vi "_SeqMgr.Code Test.vi"(11 "Module Config":T4={"Name"="SeqMgr_SW_Ver", "Parent Q"=refnum, "Is Child?"=FALSE, "Index"=0, "Dirs"={"Root"=path "", "Config"=path "C:/ATE/Config", "Logs"=path "C:/ATE/Logs", "Reports"=path "C:/ATE/Reports", "App Data"=path "C:/ProgramData/MAIN"}, "Simulate"=FALSE, "SimCtrl"=refnum}) -> ()   [LabVIEW 2024, in "EQMF.lvlib" / "SeqMgr.lvlib"]
uses:
  SeqMgr.lvlib
  SeqMgr.Result State Enum.ctl
  Module/Module Config.ctl
  Queues/Q.Element.ctl
  Module/Module.Working Dirs.ctl
  Module/Module.SW Version Info.ctl
  SeqMgr.Result Info.ctl
  Module/Window/Window.Task, Action.ctl
  Event Log/Log Action Class/Event Log.Log Params.ctl
  Event Log/Event Notification/Event Log.Log Level.ctl
  SeqMgr.lvclass
  SeqMgr.Progress Controls.ctl
  SeqMgr.Result Control Ref.ctl
  Config/Stored Controls/Class.SaveCtrls.lvclass
  Queues/Queue Utils.lvlib
  Module/Module Utils.lvlib
  Event Log/Event Log.lvlib
  Scheduler/Scheduler.lvlib
  Menu/Menu Utils.lvlib
  Config/Config Utils.lvlib
panel:
  in  "Main Tab":enum32{"Operate", "Maint"}(tab)
  in  "Default Delay ms":i32=100
  out "Simulate Indication":string="Simulating Instruments"
  out "Rev":string="v1.0.0"
  out "Test Ctrl Tab":enum32{"Idle", "Running", "Completed"}(tab)
  in  "Test Start":bool
  in  "SN":string
  out "UUT SN Status":string="Enter Operator and SN then click Start."
  out "Test Running":bool
  out "Progress":dbl(slide) scale=0.0..1.0
  in  "Test Abort":bool
  out "SN 2":string caption="SN"
  out "Failing Status":string="Failing"
  in  "Test Reset":bool
  out "SN 3":string caption="SN"
  out "Result":T2
  out "Start Time":timestamp
  out "Duration(s)":dbl format="%.2f"
  out "End Time":timestamp
  out "Current Step":string[](array[string])
  in  "Seq Steps":string[][](array[string])=[["Action1", "1000"], ["Action2", "100"], ["Action3", "500"], ["Action4", "500"]]
  out "Status":string
  in  "Stop on Fail":bool
  in  "Stop on Error":bool=TRUE
  out "Seq Name":string
  in  "Result Info":T3={"State"=enum."Passing", "Code"=0, "Description"=""}
  in  "Leave Maint":bool
  in  "SW Rev":T6={"AppName"="SeqMgr_SW_Ver", "Company"="KwestEng", "Version"="1.0", "Description"="", "PN"=""}
  # "Seq Test"
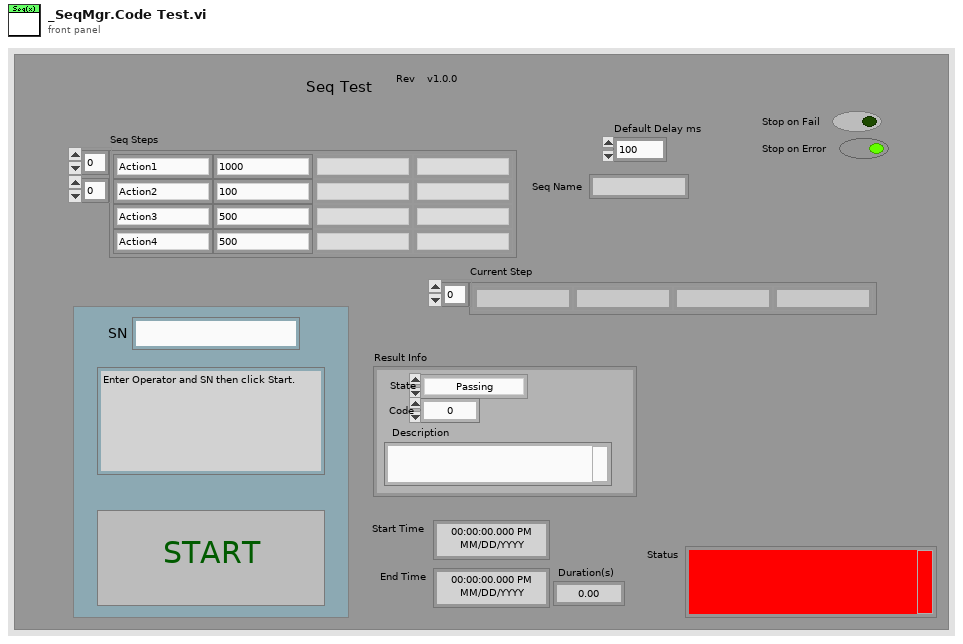
[diagram p1: front panel]
types:
  T1 = typedef "EQMF.lvlib/SeqMgr.lvlib/SeqMgr.Result State Enum.ctl" = enum16{"None", "Passing", "Failing", "PASS", "FAIL", "ABORT", "ERROR"}
  T2 = cluster{"State":T1, "Code":i32, "Description":string}
  T3 = typedef "EQMF.lvlib/SeqMgr.lvlib/SeqMgr.Result Info.ctl" = cluster{"State":T1, "Code":i32, "Description":string}
  T4 = typedef "EQMF.lvlib/Module Utils.lvlib/Module Config.ctl" = cluster{"Name":string, "Parent Q":refnum<queue>, "Is Child?":bool, "Index":i32, "Dirs":T5, "Simulate":bool, "SimCtrl":refnum<vi>}
  T5 = typedef "EQMF.lvlib/Module Utils.lvlib/Module.Working Dirs.ctl" = cluster{"Root":path, "Config":path, "Logs":path, "Reports":path, "App Data":path}
  T6 = typedef "EQMF.lvlib/Module Utils.lvlib/Module.SW Version Info.ctl" = cluster{"AppName":string, "Company":string, "Version":string, "Description":string, "PN":string}
  T7 = typedef "EQMF.lvlib/Module Utils.lvlib/Module Sys Info.ctl" = cluster{"Main Q":refnum<queue>, "Exe":bool, "SW Rev":T6, "Self Ref":refnum<vi>, "Main Tab":refnum<vi>, "Pane":refnum<vi>, "Stop":cluster{"Ref":refnum<event-registration>, "Event":refnum<user-event>}, "Cfg":T4, "Services":cluster{"Name":string, "vi ref":refnum<vi>}[], "Menu Ref":refnum<k9>, "CtrlStates":refnum<class "Class.SaveCtrls.lvclass">, "Docs":cluster{"Tags":string[], "Paths":path[]}, "Log":refnum<class "Event Notification.lvclass">, "Test Controls":refnum<vi>[], "Child Modules":cluster{"Name":string, "vi ref":refnum<vi>}[], "SW Items":string[][], "AppData":refnum<class "Class.AppData.lvclass">, "Subscriptions":refnum<class "Subscription.lvclass">, "Module Config Ref":refnum<vi>}
  T8 = enum8{"Enabled", "Disabled", "Disabled and Grayed Out"}
  T9 = typedef "EQMF.lvlib/Event Log.lvlib/Event Log.Log Params.ctl" = cluster{"Log Level":T10, "StatusTxtBoxRef":refnum<vi>, "AppID":string, "Is Child?":bool, "Parent Q":refnum<queue>}
  T10 = typedef "EQMF.lvlib/Event Log.lvlib/Event Log.Log Level.ctl" = enum16{"Normal", "Verbose", "Debug0", "Debug1", "Debug2"}
  T11 = cluster{"Child Modules":cluster{"VI Ref":refnum<vi>, "Name":string}[]}
  T12 = cluster{"Lnch":bool, string, "Status":T9, "SeqMgr":refnum<class "SeqMgr.lvclass">, "App":cluster{"Child Modules":cluster{"VI Ref":refnum<vi>, "Name":string}[]}, "Result Info":T3, "Vars":variant}
  T13 = typedef "EQMF.lvlib/SeqMgr.lvlib/SeqMgr.Result Control Ref.ctl" = cluster{"State":refnum<vi>, "Code":refnum<vi>, "Desc":refnum<vi>, "StateColors":u32[]}
  T14 = typedef "EQMF.lvlib/SeqMgr.lvlib/SeqMgr.Progress Controls.ctl" = cluster{"Running":refnum<vi>, "StartTime":refnum<vi>, "EndTime":refnum<vi>, "ProgressBar":refnum<vi>, "Duration(s)":refnum<vi>, "Test Ctrl Tab":refnum<vi>, "Failing Status":refnum<vi>}
  T15 = typedef "EQMF.lvlib/Module Utils.lvlib/Window.Task, Action.ctl" = enum16{"Resize()", "Show Panel(Bool)", "Show Scroll Bars(Bool)", "Dock to SubPanel(SubPanel Ref)", "Undock from SubPanel()", "Return to SubPanel()", "Go To Maint Tab()", "Show Maint Tab(Bool)", "Open Block Diagram()"}
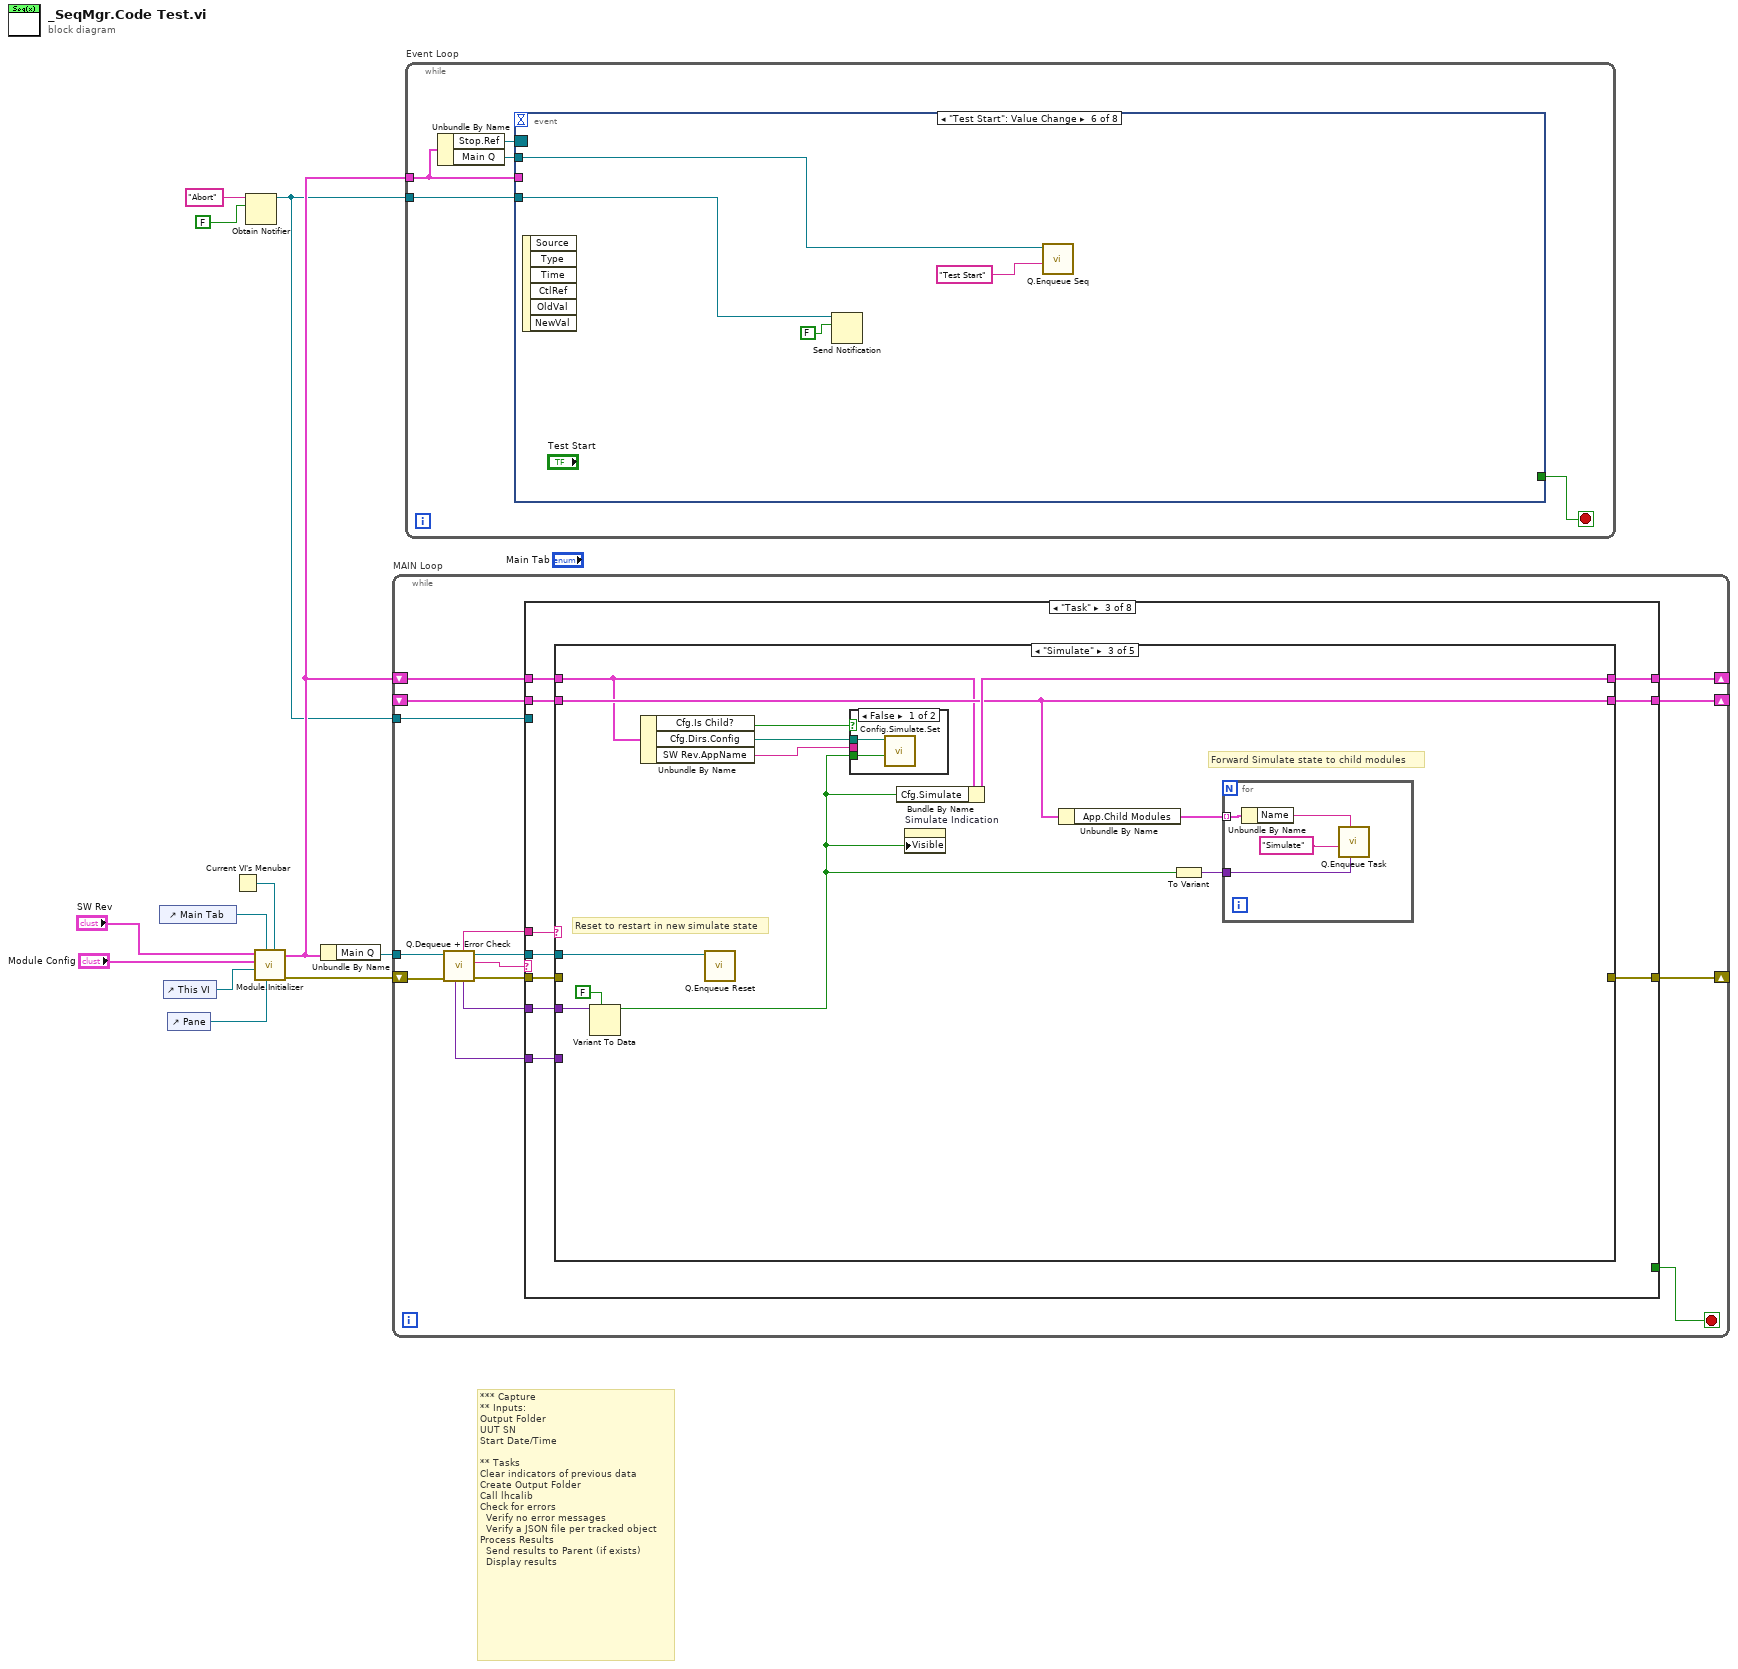
[diagram p0: block diagram]
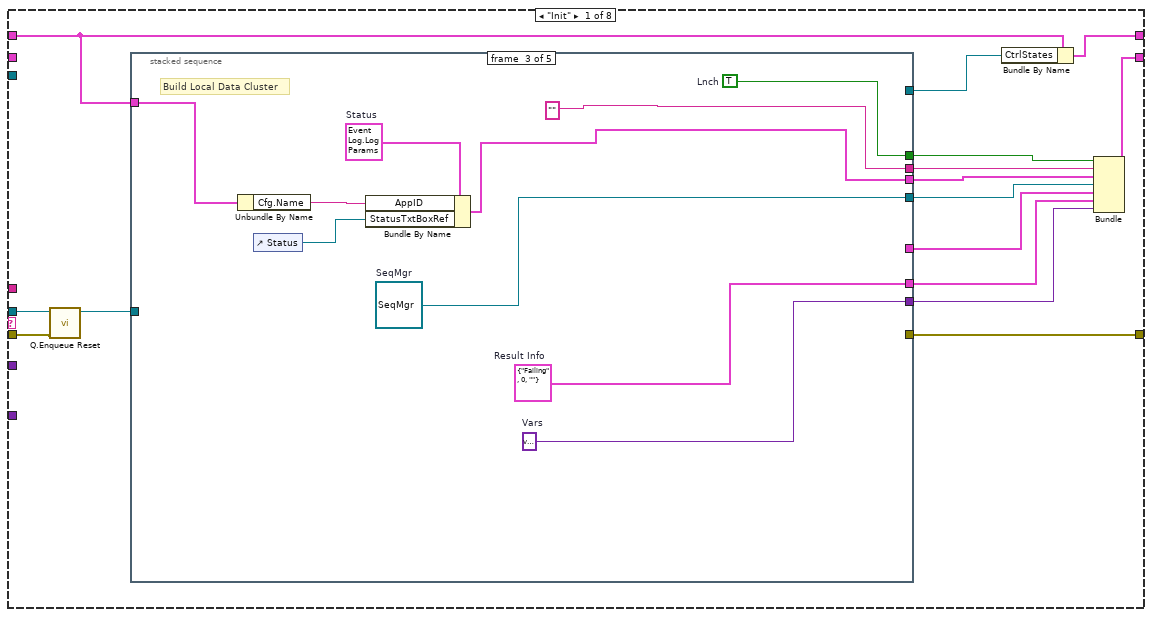
[diagram p2: hidden frame]
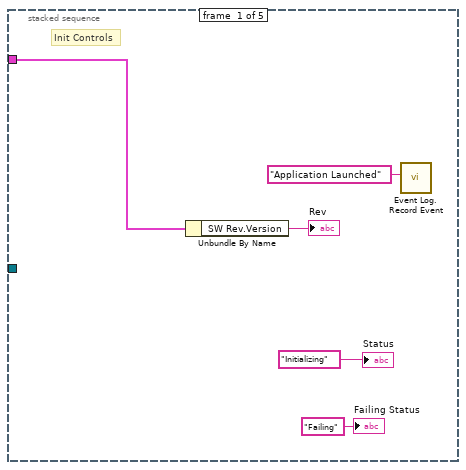
[diagram p3: hidden frame]
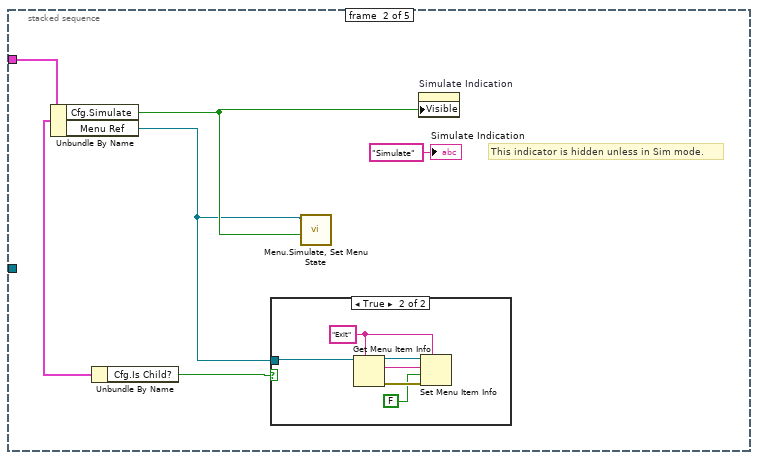
[diagram p4: hidden frame]
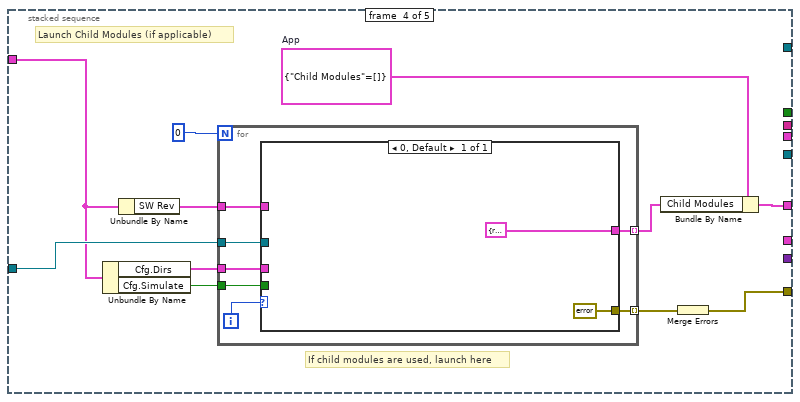
[diagram p6: hidden frame]
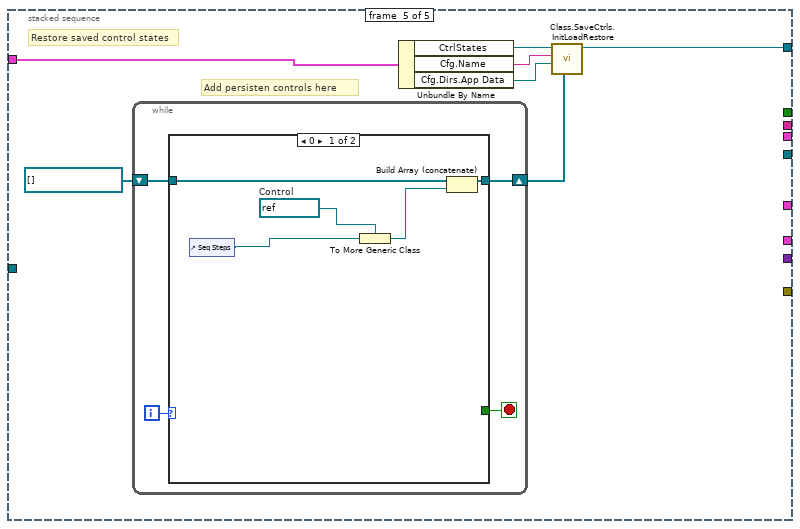
[diagram p7: hidden frame]
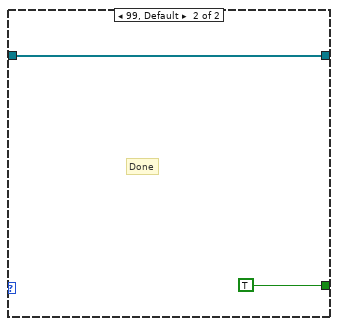
[diagram p8: hidden frame]
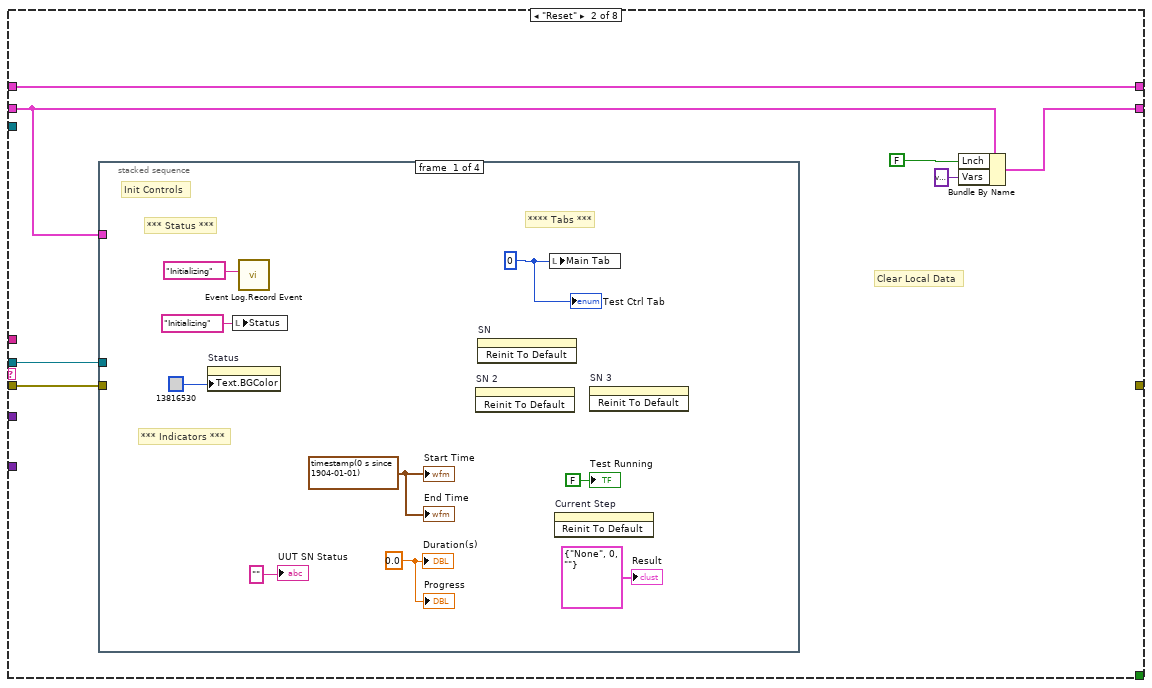
[diagram p9: hidden frame]
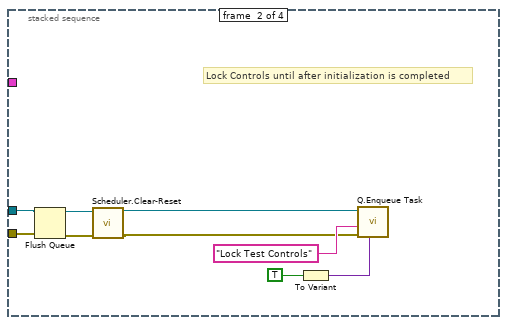
[diagram p10: hidden frame]
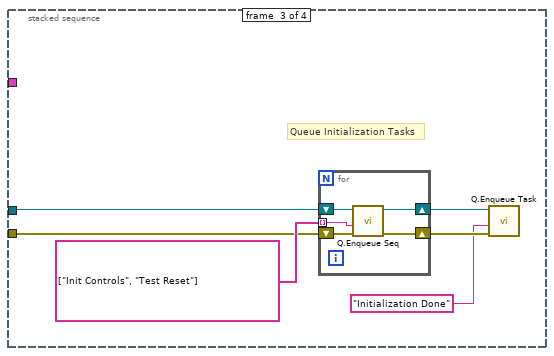
[diagram p11: hidden frame]
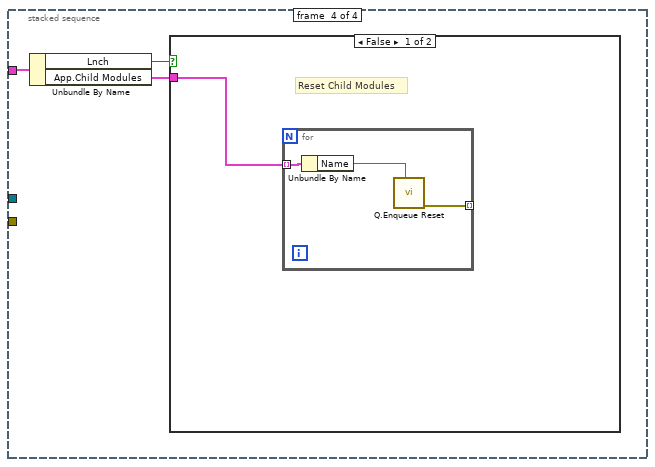
[diagram p12: hidden frame]
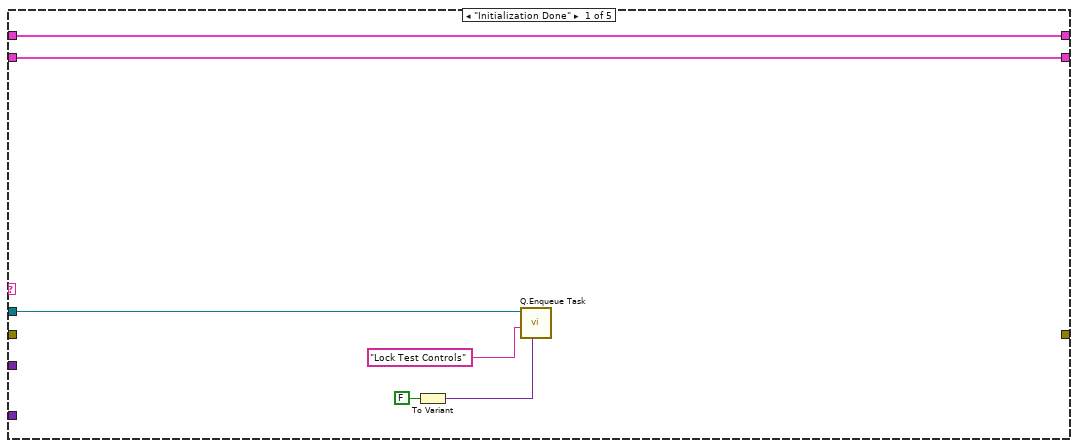
[diagram p14: hidden frame]
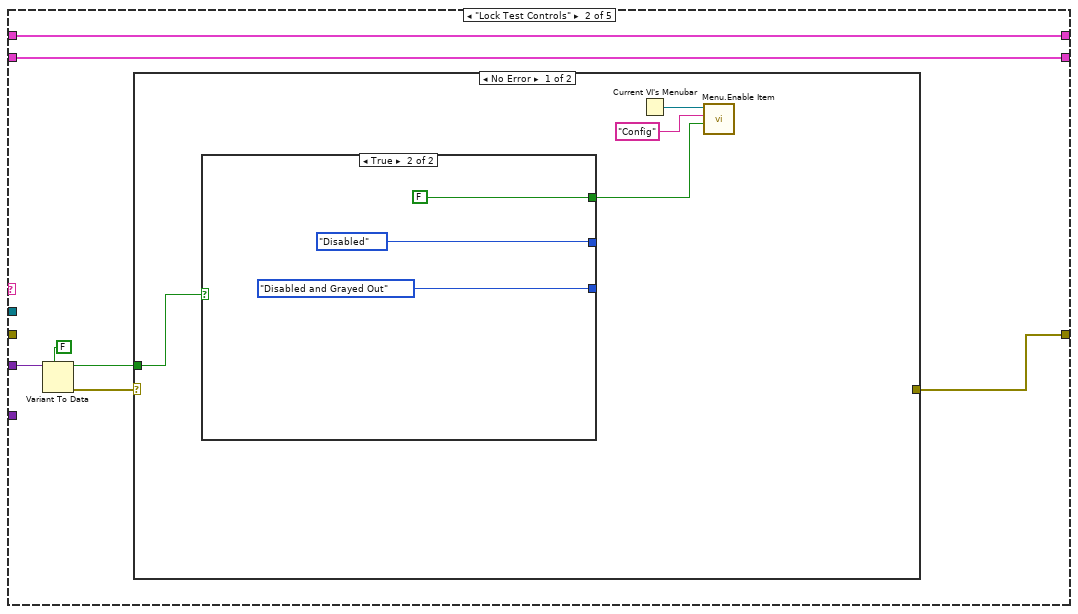
[diagram p15: hidden frame]
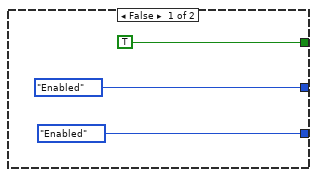
[diagram p16: hidden frame]
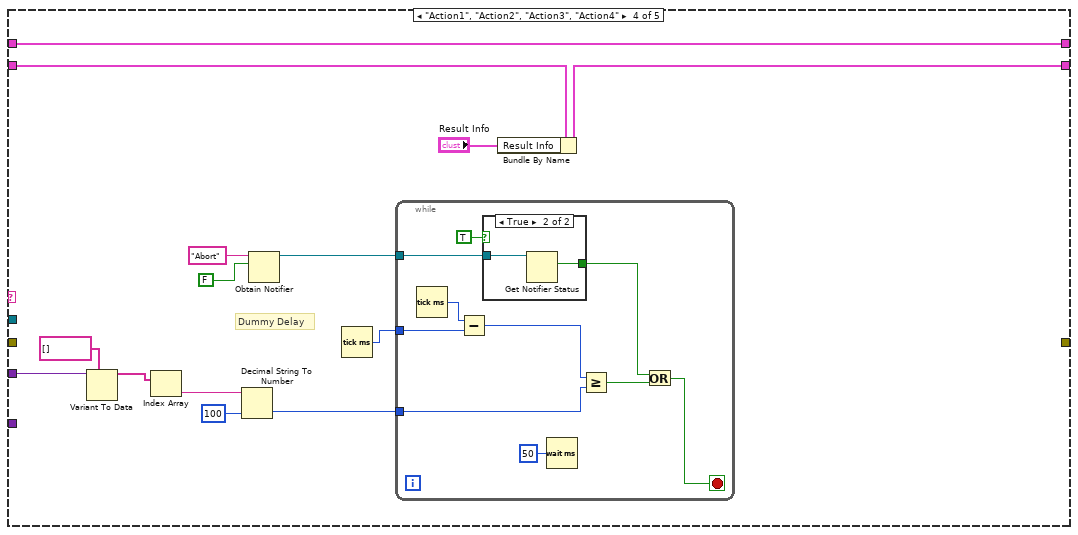
[diagram p19: hidden frame]
diagram:
  # "*** Capture\n** Inputs:\nOutput Folder\nUUT SN\nStart Date/Time\n\n** Tasks \nClear indicators of previous data\nCreate Output Folder\nCall lhcalib\nCheck for errors\n  Verify no error messages\n  Verify a JSON file per tracked object\nProcess Results\n  Send results to Parent (if exists)\n  Display results"
  n1 = control-ref of="Main Tab"() -> (w10:refnum<vi>)
  n2 = control-ref of="This VI"() -> (w9:refnum<vi>)
  n3 = control-ref of="Pane"() -> (w8:refnum<vi>)
  n4 = Current VI's Menubar() -> (w6:refnum<k9>)
  n5 = Obtain Notifier(name (unnamed)="Abort", notification data type=FALSE) -> (notifier out=w1:refnum<notifier>)  [unwired: 2 in, 2 out]
  n6 = call "Module.Initializer.vi"("Menu Ref"=w6, "Pane"=w8, "Main Tab"=w10, "Self Ref"=w9, "Module Config"="Module Config", "SW Rev"="SW Rev") -> ("error out"=w12:errorcluster, "Sys"=w7:T7)  [unwired: 4 in]
  n7 = Unbundle By Name(w7) -> ("Main Q"=w11:refnum<queue>)
  n8 = while "MAIN Loop" {
    shift-right: [w23] -> _
    shift-left: w12 -> [w21]
    shift-right: [w24] -> _
    shift-left: _ -> [w27]
    shift-right: [w25] -> _
    shift-left: w7 -> [w26]
    tunnel: w11 -> [w20]
    tunnel: w1 -> [w13]
    stop <- w15 stop-if-true
    n9 = call "Q.Dequeue + Error Check.vi"("Error In"=w21, "Q In"=w20) -> ("error out"=w22:errorcluster, "Cmd"=w19:string, "Q Out"=w18:refnum<queue>, "Data1"=w17:variant, "Sub"=w14:string, "Data2"=w16:variant)  [unwired: 4 in]
    n10 = case shown="\"Task\"" w19 {
      selector: w19 -> [_ _ _ _ _ _ w386 _]
      tunnel: w27 -> [_ w109 w158 w237 w261 w275 w388 w417]
      tunnel: w26 -> [w36 w112 w159 w238 w262 w276 w389 w418]
      tunnel: [w37 w112 w157 w236 w260 w274 w389 w418] -> w25
      tunnel: [w40 w113 w156 w235 w259 w273 w388 w417] -> w24
      tunnel: [w33 _ w150 _ w254 _ w387 w420] -> w23
      tunnel: w22 -> [w41 w110 w152 _ w255 w269 w384 _]
      tunnel: w18 -> [w42 w111 w153 w241 w256 w270 w382 _]
      tunnel: w17 -> [_ _ w154 w240 w257 w271 w385 _]
      tunnel: w16 -> [_ _ w151 w239 w253 w268 _ _]
      tunnel: w14 -> [_ _ w155 w242 w258 w272 w383 _]
      tunnel: [_ _ _ _ _ _ _ TRUE] -> w15
      tunnel: w13 -> [_ _ _ _ _ w267 _ w415]
      frame "Init" {
        n11 = call "Q.Enqueue Reset.vi"("Error In"=w41, "Q In"=w42) -> ("Q Out"=w34:refnum<queue>)  [unwired: 8 in, 1 out]
        n12 = stacked-sequence {
          tunnel: [_ _ "" _ _] -> w39
          tunnel: [_ _ w66 _ _] -> w38
          tunnel: w36 -> [w45 w49 w65 w72 w90]
          tunnel: [_ _ w63 _ _] -> w31
          tunnel: [_ _ _ _ w89] -> w35
          tunnel: [_ _ _ w78 _] -> w30
          tunnel: w34 -> [_ _ _ w73 _]
          tunnel: [_ _ _ w69 _] -> w33
          tunnel: [_ _ w68 _ _] -> w32
          tunnel: [_ _ w61 _ _] -> w29
          tunnel: [_ _ w60 _ _] -> w28
          frame #0 {
            # "Init Controls"
            n13 = Unbundle By Name(w45) -> ("SW Rev.Version"=→"Rev":string)
            n14 = call "Event Log.Record Event.vi"("Message"="Application Launched") -> ()  [unwired: 10 in, 1 out]
            "Status" <- "Initializing" ("Status")
            "Failing Status" <- "Failing" ("Failing Status")
          }
          frame #1 {
            # "This indicator is hidden unless in Sim mode."
            n15 = Unbundle By Name(w49) -> ("Cfg.Simulate"=w51:bool, "Menu Ref"=w48:refnum<k9>)
            n16 = Unbundle By Name(w49) -> ("Cfg.Is Child?"=w50:bool)
            n17 = case shown="True" w50 {
              tunnel: w48 -> [_ w54]
              frame False {
              }
              frame True {
                w56 = "Exit"
                n18 = Get Menu Item Info(7:w56, 11:w54) -> (0:w55:errorcluster, 2:w57:string, 3:w58:refnum<k9>)  [unwired: 1 in, 4 out]
                n19 = Set Menu Item Info(7:w56, 8:w55, 9:FALSE ("enabled"), 10:w57, 11:w58) -> ()  [unwired: 2 in, 2 out]
              }
            }
            n20 = call "Menu.Simulate, Set Menu State.vi"("Sim Enable"=w51, "Menu Ref"=w48) -> ()  [unwired: 8 in, 2 out]
            n21 = property on="Simulate Indication" class="Str"("Visible"=w51) -> ()  [unwired: 2 in, 2 out]
            "Simulate Indication" <- "Simulate" ("Simulate Indication")
          }
          frame #2 {
            w60 = variant  # Vars
            w61 = T3 {"State"=enum."Failing", "Code"=0, "Description"=""}  # Result Info
            w63 = refnum<class "SeqMgr.lvclass"> refnum  # SeqMgr
            w67 = T9 {"Log Level"=enum."Normal", "StatusTxtBoxRef"=refnum, "AppID"="", "Is Child?"=FALSE, "Parent Q"=refnum}  # Status
            w68 = TRUE  # Lnch
            # "Build Local Data Cluster"
            n22 = Unbundle By Name(w65) -> ("Cfg.Name"=w64:string)
            n23 = control-ref of="Status"() -> (w62:refnum<vi>)
            n24 = Bundle By Name(cluster=w67, "AppID"=w64, "StatusTxtBoxRef"=w62) -> (w66:T9)
          }
          frame #3 {
            w79 = T11 {"Child Modules"=[]}  # App
            # "If child modules are used, launch here"
            # "Launch Child Modules (if applicable)"
            n25 = Unbundle By Name(w72) -> ("Cfg.Dirs"=w75:T5, "Cfg.Simulate"=w74:bool)
            n26 = Unbundle By Name(w72) -> ("SW Rev"=w77:T6)
            n27 = for {
              N: 0 -> [_]
              tunnel: w77 -> [w86]
              tunnel: [w81] -> w71 mode=indexing
              tunnel: w73 -> [w84]
              tunnel: w75 -> [w83]
              tunnel: w74 -> [w82]
              tunnel: [w80] -> w70 mode=indexing
              i -> [w85]
              n28 = case shown="0, Default" w85 {
                tunnel: w86 -> [_]
                tunnel: w84 -> [_]
                tunnel: w83 -> [_]
                tunnel: w82 -> [_]
                tunnel: [cluster{"VI Ref":refnum<vi>, "Name":string} {"VI Ref"=refnum, "Name"=""} ("output cluster")] -> w81
                tunnel: [errorcluster {"status"=FALSE, "code"=0, "source"=""} ("error constant")] -> w80
                frame 0, Default {
                }
              }
            }
            n29 = Bundle By Name(cluster=w79, "Child Modules"=w71) -> (w78:T11)
            n30 = Merge Errors(w70) -> (w69:errorcluster)
          }
          frame #4 {
            # "Add persisten controls here"
            # "Restore saved control states"
            n31 = while {
              shift-right: [w97] -> w91
              shift-left: refnum<vi>[] [] -> [w98]
              i -> [w99]
              stop <- w96 stop-if-true
              n32 = case shown="0" w99 {
                tunnel: w98 -> [w103 w106]
                tunnel: [w104 w106] -> w97
                tunnel: [_ TRUE] -> w96
                frame 0 {
                  w101 = refnum<vi> refnum  # Control
                  n33 = control-ref of="Seq Steps"() -> (w100:refnum<vi>)
                  n34 = To More Generic Class(target class=w101, reference=w100) -> (generic class reference=w102:refnum<vi>)
                  n35 = Build Array (concatenate)(w103, w102) -> (w104:refnum<vi>[])
                }
                frame 99, Default {
                  # "Done"
                }
              }
            }
            n36 = Unbundle By Name(w90) -> ("CtrlStates"=w92:refnum<class "Class.SaveCtrls.lvclass">, "Cfg.Name"=w94:string, "Cfg.Dirs.App Data"=w93:path)
            n37 = call-dynamic "Class.SaveCtrls.InitLoadRestore.vi"("Ctrl Array"=w91, "Module Data Dir"=w93, "Module Name"=w94, "CtrlStates In"=w92) -> ("CtrlStates"=w89:refnum<class "Class.SaveCtrls.lvclass">)  [unwired: 6 in, 1 out]
          }
        }
        n38 = Bundle By Name(cluster=w36, "CtrlStates"=w35) -> (w37:T7)
        n39 = Bundle("Lnch"=w32, w39, "Status"=w38, "SeqMgr"=w31, "App"=w30, "Result Info"=w29, "Vars"=w28) -> (w40:T12)  [unwired: 1 in]
      }
      frame "Reset" {
        # "Clear Local Data"
        n40 = stacked-sequence {
          tunnel: w111 -> [_ w124 w132 _]
          tunnel: w110 -> [_ w123 w136 _]
          tunnel: w109 -> [_ _ _ w145]
          frame #0 {
            w118 = timestamp(0 s since 1904-01-01) ("End Time")
            w117 = 0.0 ("Duration(s)")
            w119 = 0
            # "*** Indicators ***"
            # "**** Tabs ***"
            # "*** Status ***"
            # "Init Controls"
            n41 = property on="Status" class="Str"("Text.BGColor"=u32 13816530) -> ()  [unwired: 2 in, 2 out]
            n42 = local write "Status"("Initializing" ("Status")) -> ()
            n43 = call "Event Log.Record Event.vi"("Message"="Initializing") -> ()  [unwired: 10 in, 1 out]
            n44 = invoke on="SN 2" class="Str" method="Reinit To Default"() -> ()  [unwired: 3 in, 3 out]
            n45 = invoke on="SN" class="Str" method="Reinit To Default"() -> ()  [unwired: 3 in, 3 out]
            n46 = local write "Main Tab"(w119) -> ()
            n47 = invoke on="Current Step" class="Arr (strict)" method="Reinit To Default"() -> ()  [unwired: 3 in, 3 out]
            n48 = invoke on="SN 3" class="Str" method="Reinit To Default"() -> ()  [unwired: 3 in, 3 out]
            "Test Ctrl Tab" <- w119
            "Duration(s)" <- w117
            "Start Time" <- w118
            "End Time" <- w118
            "Progress" <- w117
            "Test Running" <- FALSE ("Test Running")
            "Result" <- T2 {"State"=enum."None", "Code"=0, "Description"=""} ("Result")
            "UUT SN Status" <- ""
          }
          frame #1 {
            # "Lock Controls until after initialization is completed"
            n49 = Flush Queue(queue=w124, error in (no error)=w123) -> (queue out=w125:refnum<queue>, error out=w128:errorcluster)  [unwired: 1 out]
            n50 = call "Scheduler.Clear-Reset.vi"("error in"=w128, "Q In"=w125) -> ("error out"=w126:errorcluster, "Q Out"=w127:refnum<queue>)  [unwired: 8 in]
            n51 = To Variant(anything=TRUE) -> (Variant=w130:variant)
            n52 = call "Q.Enqueue Task.vi"("Data1"=w130, "Error In"=w126, "Task Name"="Lock Test Controls", "Q In"=w127) -> ()  [unwired: 6 in, 2 out]
          }
          frame #2 {
            # "Queue Initialization Tasks"
            n53 = for {
              shift-right: [w140] -> w134
              shift-left: w136 -> [w141]
              tunnel: string[] ["Init Controls", "Test Reset"] -> [w138] mode=indexing
              shift-right: [w139] -> w135
              shift-left: w132 -> [w142]
              n54 = call "Q.Enqueue Seq.vi"("Error In"=w141, "Seq Task Name"=w138, "Q In"=w142) -> ("error out"=w140:errorcluster, "Q Out"=w139:refnum<queue>)  [unwired: 7 in]
            }
            n55 = call "Q.Enqueue Task.vi"("Error In"=w134, "Task Name"="Initialization Done", "Q In"=w135) -> ()  [unwired: 7 in, 2 out]
          }
          frame #3 {
            n56 = Unbundle By Name(w145) -> ("Lnch"=w144:bool, "App.Child Modules"=w143:cluster{"VI Ref":refnum<vi>, "Name":string}[])
            n57 = case shown="False" w144 {
              tunnel: w143 -> [w146 _]
              frame False {
                # "Reset Child Modules"
                n58 = for {
                  tunnel: w146 -> [w149] mode=indexing
                  tunnel: [w147] -> _ mode=indexing
                  n59 = Unbundle By Name(w149) -> ("Name"=w148:string)
                  n60 = call "Q.Enqueue Reset.vi"("Q Name"=w148) -> ("error out"=w147:errorcluster)  [unwired: 9 in, 1 out]
                }
              }
              frame True {
                # "Do not reset at launch.\nThey are already reset"
              }
            }
          }
        }
        n61 = Bundle By Name(cluster=w109, "Lnch"=FALSE ("Test.Running"), "Vars"=variant) -> (w113:T12)
      }
      frame "Task" {
        n62 = case shown="\"Simulate\"" w155 {
          selector: w155 -> [_ _ _ _ w232]
          tunnel: w159 -> [w165 w172 w188 w215 w233]
          tunnel: w158 -> [w160 w171 w192 w209 w234]
          tunnel: [w165 w172 w193 w215 w233] -> w157
          tunnel: [w160 w171 w192 w208 w234] -> w156
          tunnel: w154 -> [_ w170 w195 w214 w231]
          tunnel: w153 -> [w164 _ w189 _ _]
          tunnel: w152 -> [_ _ _ _ w229]
          tunnel: w151 -> [_ _ _ _ w230]
          tunnel: [_ w166 _ _ w228] -> w150
          frame "Initialization Done" {
            n63 = To Variant(anything=FALSE) -> (Variant=w162:variant)
            n64 = call "Q.Enqueue Task.vi"("Data1"=w162, "Task Name"="Lock Test Controls", "Q In"=w164) -> ()  [unwired: 7 in, 2 out]
          }
          frame "Lock Test Controls" {
            n65 = Variant To Data(type=FALSE, Variant=w170) -> (data=w167:bool, error out=w168:errorcluster)  [unwired: 1 in]
            n66 = case shown="No Error" w168 {
              selector: w168 -> [_ w183]
              tunnel: w167 -> [w176 _]
              tunnel: [_ w183] -> w166
              frame No Error {
                n67 = case shown="True" w176 {
                  tunnel: [T8."Enabled" ("Disabled") T8."Disabled and Grayed Out" ("Disabled")] -> _
                  tunnel: [T8."Enabled" ("Disabled") T8."Disabled" ("Disabled")] -> _
                  tunnel: [TRUE ("Enable") FALSE ("Enable")] -> w173
                  frame False {
                  }
                  frame True {
                  }
                }
                n68 = Current VI's Menubar() -> (w174:refnum<k9>)
                n69 = call "Menu.Enable Item.vi"("Enable"=w173, "Tag"="Config", "Menu Ref"=w174) -> ()  [unwired: 7 in, 2 out]
              }
              frame Error {
              }
            }
          }
          frame "Simulate" {
            # "Reset to restart in new simulate state"
            # "Forward Simulate state to child modules"
            n70 = Variant To Data(type=FALSE, Variant=w195) -> (data=w185:bool)  [unwired: 1 in, 1 out]
            n71 = Unbundle By Name(w188) -> ("Cfg.Is Child?"=w184:bool, "Cfg.Dirs.Config"=w187:path, "SW Rev.AppName"=w186:string)
            n72 = call "Q.Enqueue Reset.vi"("Q In"=w189) -> ()  [unwired: 9 in, 2 out]
            n73 = case shown="False" w184 {
              tunnel: w187 -> [w197 _]
              tunnel: w186 -> [_ _]
              tunnel: w185 -> [w196 _]
              frame False {
                n74 = call "Config.Simulate.Set.vi"("Simulate"=w196, "Config Folder"=w197) -> ()  [unwired: 9 in, 1 out]
              }
              frame True {
              }
            }
            n75 = Bundle By Name(cluster=w188, "Cfg.Simulate"=w185) -> (w193:T7)
            n76 = property on="Simulate Indication" class="Str"("Visible"=w185) -> ()  [unwired: 2 in, 2 out]
            n77 = Unbundle By Name(w192) -> ("App.Child Modules"=w191:cluster{"VI Ref":refnum<vi>, "Name":string}[])
            n78 = To Variant(anything=w185) -> (Variant=w190:variant)
            n79 = for {
              tunnel: w191 -> [w201] mode=indexing
              tunnel: w190 -> [w198]
              n80 = Unbundle By Name(w201) -> ("Name"=w200:string)
              n81 = call "Q.Enqueue Task.vi"("Data1"=w198, "Q Name"=w200, "Task Name"="Simulate") -> ()  [unwired: 7 in, 2 out]
            }
          }
          frame "Action1", "Action2", "Action3", "Action4" {
            # "Dummy Delay"
            n82 = Variant To Data(type=string[] [], Variant=w214) -> (data=w212:string[])  [unwired: 1 in, 1 out]
            n83 = Index Array(array=w212) -> (element=w211:string)  [unwired: 1 in]
            n84 = Decimal String To Number(string=w211, default (0L)=u32 100 ("milliseconds to wait")) -> (number=w203:u32)  [unwired: 1 in, 1 out]
            n85 = Obtain Notifier(name (unnamed)="Abort", notification data type=FALSE) -> (notifier out=w205:refnum<notifier>)  [unwired: 2 in, 2 out]
            n86 = Tick Count (ms)() -> (millisecond timer value=w202:u32)
            n87 = while {
              tunnel: w205 -> [w225]
              tunnel: w203 -> [w224]
              tunnel: w202 -> [w219]
              stop <- w221 stop-if-true
              n88 = Tick Count (ms)() -> (millisecond timer value=w220:u32)
              n89 = Subtract(x=w220, y=w219) -> (x-y=w217:u32)
              n90 = case shown="True" TRUE {
                tunnel: w225 -> [_ w227]
                tunnel: [_ w226] -> w222
                frame False {
                }
                frame True {
                  n91 = Get Notifier Status(notifier=w227) -> (current notification=w226:bool)  [unwired: 1 in, 4 out]
                }
              }
              n92 = Wait (ms)(milliseconds to wait=u32 50) -> ()  [unwired: 1 out]
              n93 = Greater Or Equal?(x=w217, y=w224) -> (x >= y?=w223:bool)
              n94 = Or(x=w222, y=w223) -> (x .or. y?=w221:bool)
            }
            n95 = Bundle By Name(cluster=w209, "Result Info"="Result Info") -> (w208:T12)
          }
          frame Default {
            n96 = call "Module.Default Tasks.vi"("Sys"=w233, "error in"=w229, "Data2"=w230, "Data1"=w231, "Sub"=w232) -> ("error out"=w228:errorcluster)  [unwired: 5 in, 1 out]
          }
        }
      }
      frame "App" {
        n97 = case shown="\"Set Logging Level\"" w242 {
          tunnel: w241 -> [_ _]
          tunnel: w240 -> [_ w247]
          tunnel: w239 -> [_ _]
          tunnel: w238 -> [w244 w250]
          tunnel: w237 -> [w243 w249]
          tunnel: [w244 w250] -> w236
          tunnel: [w243 w248] -> w235
          frame Default {
          }
          frame "Set Logging Level" {
            n98 = Variant To Data(type=0, Variant=w247) -> (data=w245:i32)  [unwired: 1 in, 1 out]
            n99 = Bundle By Name(cluster=w249, "Status.Log Level"=w245) -> (w248:T12)
          }
        }
      }
      frame "Function" {
        n100 = case shown="Default" w258 {
          tunnel: w262 -> [w265]
          tunnel: w261 -> [w266]
          tunnel: [w265] -> w260
          tunnel: [w266] -> w259
          tunnel: w257 -> [_]
          tunnel: w256 -> [_]
          tunnel: w255 -> [w263]
          tunnel: w253 -> [_]
          tunnel: [w263] -> w252
          tunnel: [variant] -> w251
          frame Default {
            # "Do nothing.  The sender of the command will report an error (timeout or incorrect data)."
          }
        }
        n101 = call "Q.Return Function Data.vi"("error in"=w252, "Data2"=w253, "Ret Data"=w251) -> ("error out"=w254:errorcluster)  [unwired: 8 in]
      }
      frame "Seq" {
        n102 = case shown="\"Test Start\"" w272 {
          tunnel: w276 -> [w295 w324 w341 w367 w373 w378 w380]
          tunnel: w275 -> [w292 w316 w338 w364 w372 w376 w381]
          tunnel: [w295 w324 w341 w367 w373 w378 w380] -> w274
          tunnel: [w291 w323 w329 w363 w372 w377 w381] -> w273
          tunnel: w271 -> [_ _ _ _ _ _ _]
          tunnel: w270 -> [_ w299 w336 _ w368 _ _]
          tunnel: w269 -> [_ _ _ _ _ _ w379]
          tunnel: w268 -> [_ _ _ _ _ _ _]
          tunnel: [_ _ _ _ _ _ w379] -> _
          tunnel: w267 -> [_ _ _ _ _ _ _]
          frame "Init Controls" {
            w283 = T13 {"State"=refnum, "Code"=refnum, "Desc"=refnum, "StateColors"=[13816530, 11009952, 16758968, 6618880, 16711680, 16711680, 16711680]}  # ResultCtrls
            w290 = T14 {"Running"=refnum, "StartTime"=refnum, "EndTime"=refnum, "ProgressBar"=refnum, "Duration(s)"=refnum, "Test Ctrl Tab"=refnum, "Failing Status"=refnum}  # ProgressCtrls
            n103 = control-ref of="Failing Status"() -> (w277:refnum<vi>)
            n104 = control-ref of="Progress"() -> (w285:refnum<vi>)
            n105 = control-ref of="Test Ctrl Tab"() -> (w289:refnum<vi>)
            n106 = control-ref of="Duration(s)"() -> (w284:refnum<vi>)
            n107 = control-ref of="Test Running"() -> (w288:refnum<vi>)
            n108 = control-ref of="Start Time"() -> (w287:refnum<vi>)
            n109 = control-ref of="End Time"() -> (w286:refnum<vi>)
            n110 = control-ref of="Description"() -> (w280:refnum<vi>)
            n111 = control-ref of="Code"() -> (w281:refnum<vi>)
            n112 = control-ref of="State"() -> (w282:refnum<vi>)
            n113 = Bundle By Name(cluster=w290, "Running"=w288, "StartTime"=w287, "EndTime"=w286, "ProgressBar"=w285, "Duration(s)"=w284, "Test Ctrl Tab"=w289, "Failing Status"=w277) -> (w279:T14)
            n114 = Unbundle By Name(w292) -> ("SeqMgr"=w294:refnum<class "SeqMgr.lvclass">)
            n115 = Bundle By Name(cluster=w283, "State"=w282, "Code"=w281, "Desc"=w280) -> (w278:T13)
            n116 = call "SeqMgr.Initialize Seq, Init Progress Controls.vi"("ResultCtrls"=w278, "ProgressCtrls"=w279, "SeqMgr in"=w294) -> ("SeqMgr out"=w293:refnum<class "SeqMgr.lvclass">)  [unwired: 7 in, 1 out]
            n117 = Bundle By Name(cluster=w292, "SeqMgr"=w293) -> (w291:T12)
          }
          frame "Test Start" {
            w314 = "Test Start"
            n118 = To Variant(anything=TRUE) -> (Variant=w302:variant)
            n119 = Unbundle By Name(w316) -> ("Status"=w315:T9)
            n120 = call "Q.Enqueue Task.vi"("Data1"=w302, "Task Name"="Lock Test Controls", "Q In"=w299) -> ("Q Out"=w298:refnum<queue>)  [unwired: 7 in, 1 out]
            n121 = call "Q.Enqueue Seq.vi"("Seq Task Name"="Test Running" ("Task Name"), "Q In"=w298) -> ()  [unwired: 8 in, 2 out]
            n122 = call "Event Log.Record Status Message and Even.vi"("Status Msg"=w314, "Event Log"=w314, "Status"=w315) -> ()  [unwired: 8 in, 1 out]
            n123 = Unbundle By Name(w316) -> ("SeqMgr"=w322:refnum<class "SeqMgr.lvclass">)
            n124 = call "SeqMgr.Set Test Stop Criteria.vi"("Stop on Error"="Stop on Error", "Stop on Fail"="Stop on Fail", "SeqMgr in"=w322) -> ("SeqMgr out"=w313:refnum<class "SeqMgr.lvclass">)  [unwired: 7 in, 1 out]
            n125 = Number To Decimal String(number="Default Delay ms") -> (decimal integer string=w310:string)  [unwired: 1 in]
            n126 = Build Array("Delay_ms", w310) -> (w307:string[])
            n127 = Build Array("SN", "SN") -> (w306:string[])
            n128 = Build Array(w307, w306) -> (w305:string[][])
            n129 = call "SeqMgr.Variables - Add, Replace.vi"("Name, Value"=w305, "Init"=TRUE, "SeqMgr in"=w313) -> ("SeqMgr out"=w303:refnum<class "SeqMgr.lvclass">)  [unwired: 7 in, 1 out]
            n130 = call "SeqMgr.Start Sequence.vi"("SeqSteps"="Seq Steps", "SeqMgr in"=w303) -> ("Name"=→"Seq Name":string, "SeqMgr out"=w318:refnum<class "SeqMgr.lvclass">)  [unwired: 6 in, 2 out]
            n131 = Bundle By Name(cluster=w316, "Result Info"=T3 {"State"=enum."Passing", "Code"=0, "Description"=""}, "SeqMgr"=w318) -> (w323:T12)
            "SN 2" <- "SN"
            "SN 3" <- "SN"
          }
          frame "Test Running" {
            n132 = Unbundle By Name(w338) -> ("SeqMgr"=w340:refnum<class "SeqMgr.lvclass">, "Result Info"=w327:T3)
            n133 = call "SeqMgr.Update Progress.vi"("Result Info"=w327, "SeqMgr in"=w340) -> ("Result Info Out"=w326:T3, "Test State"=w332:enum32{"Idle", "Running", "Completed"}, "SeqMgr out"=w339:refnum<class "SeqMgr.lvclass">, "New Step"=w325:string[])  [unwired: 3 in, 3 out]
            "Current Step" <- w325
            n134 = Delete From Array(array=w325, index=0) -> (deleted portion=w337:string, array with subset deleted=w335:string[])  [unwired: 1 in]
            n135 = To Variant(anything=w335) -> (Variant=w334:variant)
            n136 = case shown="\"Running\"" w332 {
              tunnel: w337 -> [_ w346 _]
              tunnel: w336 -> [_ w351 w358]
              tunnel: w334 -> [_ w350 _]
              tunnel: ["Idle" w345 w354] -> w330
              tunnel: w326 -> [_ _ w355]
              tunnel: [u32 13816530 ("Status Color(Lt Grey)") u32 13816530 ("Status Color(Lt Grey)") w352] -> w328
              frame "Idle", Default {
                # "Do Nothing"
              }
              frame "Running" {
                n137 = call "Q.Enqueue Task.vi"("Data1"=w350, "Task Name"=w346, "Q In"=w351) -> ("Q Out"=w348:refnum<queue>)  [unwired: 7 in, 1 out]
                n138 = Format Into String(format string="Test Step: %s", w346) -> (resulting string=w345:string)  [unwired: 2 in, 1 out]
                n139 = call "Q.Enqueue Seq.vi"("Seq Task Name"="Test Running", "Q In"=w348) -> ()  [unwired: 8 in, 2 out]
              }
              frame "Completed" {
                n140 = Unbundle By Name(w355) -> ("State"=w353:T1)
                n141 = call "Q.Enqueue Seq.vi"("Seq Task Name"="Test Completed", "Q In"=w358) -> ()  [unwired: 8 in, 2 out]
                n142 = Format Into String(format string="Test Completed: %s" ("Seq Task Name"), w353) -> (resulting string=w354:string)  [unwired: 2 in, 1 out]
                n143 = case shown="\"None\"" w353 {
                  tunnel: [u32 13816530 ("Status Color(Lt Grey)") u32 6618880 ("Status Color(Lt Grey)") u32 16711680 ("Status Color(Lt Grey)")] -> w352
                  frame "None" {
                  }
                  frame "Passing", "PASS" {
                  }
                  frame "Failing", Default {
                  }
                }
              }
            }
            n144 = Bundle By Name(cluster=w338, "SeqMgr"=w339) -> (w329:T12)
            n145 = Unbundle By Name(w329) -> ("Status"=w331:T9)
            n146 = call "Event Log.Record Status Message and Even.vi"("Status Color(Lt Grey)"=w328, "Status Msg"=w330, "Event Log"=w330, "Status"=w331) -> ()  [unwired: 7 in, 1 out]
          }
          frame "Test Abort" {
            n147 = Bundle By Name(cluster=w364, "Result Info.State"=SeqMgr.Result_State_Enum."ABORT" ("State"), "Result Info.Code"=-1 ("Code"), "Result Info.Description"="Test aborted by operator.") -> (w363:T12)
          }
          frame "Test Completed" {
            n148 = To Variant(anything=FALSE) -> (Variant=w371:variant)
            n149 = call "Q.Enqueue Task.vi"("Data1"=w371, "Task Name"="Lock Test Controls", "Q In"=w368) -> ()  [unwired: 7 in, 2 out]
          }
          frame "Test Reset" {
            n150 = Unbundle By Name(w376) -> ("SeqMgr"=w374:refnum<class "SeqMgr.lvclass">)
            n151 = invoke on="SN" class="Str" method="Reinit To Default"() -> ()  [unwired: 3 in, 3 out]
            n152 = call "SeqMgr.Test Reset.vi"("SeqMgr in"=w374) -> ("SeqMgr out"=w375:refnum<class "SeqMgr.lvclass">)  [unwired: 9 in, 1 out]
            n153 = Bundle By Name(cluster=w376, "SeqMgr"=w375) -> (w377:T12)
          }
          frame Default {
          }
        }
      }
      frame "Error", Default {
        n154 = case shown="\"Error\"" w386 {
          selector: w386 -> [_ w408]
          tunnel: [w391 w409] -> w387
          tunnel: w385 -> [w397 _]
          tunnel: w384 -> [w395 _]
          tunnel: w383 -> [w396 _]
          tunnel: w382 -> [w393 _]
          frame "Error" {
            n155 = case shown="\"Error\"" w396 {
              tunnel: w397 -> [_ w407]
              tunnel: w395 -> [w403 _]
              tunnel: [w403 w405] -> w390
              tunnel: w393 -> [w402 w404]
              tunnel: [w402 w404] -> w392
              frame Default {
              }
              frame "Error" {
                n156 = Variant To Data(type=errorcluster {"status"=FALSE, "code"=0, "source"=""} ("error constant"), Variant=w407) -> (data=w405:errorcluster)  [unwired: 1 in, 1 out]
              }
            }
            n157 = call "Dialogx.Error Message.vi"("error in"=w390) -> ("Selection"=w394:enum16{"Exit", "Reset", "Ignore"})
            n158 = call "Event Log.Record Event.vi"("error in"=w390) -> ()  [unwired: 10 in, 1 out]
            n159 = case shown="\"Reset\"" w394 {
              tunnel: w392 -> [w399 _ w401]
              tunnel: [w398 _ w400] -> w391
              frame "Exit", Default {
                n160 = call "Q.Enqueue Exit.vi"("Q In"=w399) -> ("error out"=w398:errorcluster)  [unwired: 9 in, 1 out]
              }
              frame "Ignore" {
              }
              frame "Reset" {
                n161 = call "Q.Enqueue Reset.vi"("Q In"=w401) -> ("error out"=w400:errorcluster)  [unwired: 9 in, 1 out]
              }
            }
          }
          frame Default {
            n162 = Concatenate Strings("Undefined State: \"", w408, "\".") -> (w410:string)
            n163 = Bundle By Name(cluster=errorcluster {"status"=TRUE, "code"=-5000, "source"=""} ("error constant"), "source"=w410) -> (w409:errorcluster)
          }
        }
      }
      frame "Exit" {
        # "This connection is made to not close\n the module until exit tasks are done."
        n164 = stacked-sequence {
          tunnel: w417 -> [_ w422]
          tunnel: [errorcluster {"status"=FALSE, "code"=0, "source"=""} ("error constant") _] -> w416
          frame #0 {
            # "Close connection to instruments"
          }
          frame #1 {
            # "Leave error not connected\nIgnore errors"
            # "Send Exit command to child modules"
            n165 = Unbundle By Name(w422) -> ("App.Child Modules"=w423:cluster{"VI Ref":refnum<vi>, "Name":string}[])
            n166 = for {
              tunnel: w423 -> [w426] mode=indexing
              tunnel: [w424] -> _ mode=indexing
              n167 = Unbundle By Name(w426) -> ("Name"=w425:string)
              n168 = call "Q.Enqueue Exit.vi"("Q Name"=w425) -> ("error out"=w424:errorcluster)  [unwired: 9 in, 1 out]
            }
          }
        }
        n169 = Release Notifier(notifier=w415, force destroy? (F)=TRUE) -> ()  [unwired: 1 in, 3 out]
        n170 = call "Module.Destructor.vi"("error in"=w416, "Sys"=w418) -> ("error out"=w420:errorcluster)  [unwired: 9 in]
      }
    }
  }
  n171 = while "Event Loop" {
    tunnel: w7 -> [w430]
    tunnel: w1 -> [w427]
    stop <- w431 stop-if-true
    n172 = Unbundle By Name(w430) -> ("Stop.Ref"=w429:refnum<event-registration>, "Main Q"=w428:refnum<queue>)
    n173 = event shown="[5] \"Test Start\": Value Change" {
      selector: w429 -> [_ _ _ _ _ _ _ _]
      dyn-events: _ -> [_ _ _ _ _ _ _ _]
      timeout: _ -> [_ _ _ _ _ _ _ _]
      tunnel: [w434 _ _ w452 TRUE _ _ _] -> w431
      tunnel: w430 -> [w433 _ _ w450 _ _ _ _]
      tunnel: w428 -> [w436 w446 _ w451 _ w476 w481 w483]
      tunnel: w427 -> [_ _ _ _ _ w474 w479 _]
      event Panel Close? {
        n174 = event-data() -> ()  [unwired: 1 in, 4 out]
        n175 = Unbundle By Name(w433) -> ("Cfg.Is Child?"=w432:bool)
        n176 = case shown="True" w432 {
          tunnel: w436 -> [w439 w442]
          tunnel: [TRUE TRUE] -> w435
          tunnel: [TRUE FALSE] -> w434
          tunnel: [_ w440] -> _
          frame False {
            # "Parent - Exit"
            n177 = call "Q.Enqueue Exit.vi"("Q In"=w439) -> ()  [unwired: 9 in, 2 out]
          }
          frame True {
            # "Child - Hide Panel and if was \nin a subpanel, return to subpanel."
            n178 = call "Module.Window, Q Task.vi"("Action"=Window.Task,_Action."Return to SubPanel()", "Q In"=w442) -> ("error out"=w440:errorcluster)  [unwired: 8 in, 1 out]
          }
        }
        n179 = event-data("Discard?"=w435) -> ()  [unwired: 1 in, 1 out]
      }
      event Panel Resize {
        n180 = event-data() -> ()  [unwired: 1 in, 8 out]
        n181 = call "Module.Window, Q Task.vi"("Action"=Window.Task,_Action."Resize()", "Q In"=w446) -> ()  [unwired: 8 in, 2 out]
      }
      event "Leave Maint": Value Change {
        n182 = event-data() -> ()  [unwired: 1 in, 6 out]
        n183 = local write "Main Tab"(0) -> ()
      }
      event Menu Selection (User) {
        n184 = event-data() -> ("MenuRef"=w448:refnum<k9>, "ItemTag"=w449:string)  [unwired: 1 in, 5 out]
        n185 = case shown="\"Help.About\"" w449 {
          selector: w449 -> [w454 _ _ _ _ w464 _ _]
          tunnel: [_ TRUE _ _ _ _ _ _] -> w452
          tunnel: w451 -> [_ w457 _ w460 _ w468 w470 w472]
          tunnel: [_ _ w459 _ _ _ _ _] -> _
          tunnel: w450 -> [w453 _ _ _ w462 _ _ _]
          tunnel: w448 -> [_ _ _ _ _ w465 _ _]
          frame Default {
            # "Check if a help document was selected.\nIf so, open the document"
            n186 = Unbundle By Name(w453) -> ("Docs.Tags"=w456:string[], "Docs.Paths"=w455:path[])
            n187 = call "Menu.Help, Open User Manual Items.vi"("Menu Tag Selection"=w454, "Paths"=w455, "Tags"=w456) -> ()  [unwired: 8 in, 1 out]
          }
          frame "Exit" {
            n188 = call "Q.Enqueue Exit.vi"("Q In"=w457) -> ()  [unwired: 9 in, 2 out]
          }
          frame "Event Log" {
            n189 = call "Event Log.Show.vi"() -> ("error out"=w459:errorcluster)  [unwired: 11 in]
          }
          frame "Reset" {
            n190 = call "Q.Enqueue Reset.vi"("Q In"=w460) -> ()  [unwired: 9 in, 2 out]
          }
          frame "Help.About" {
            n191 = Unbundle By Name(w462) -> ("SW Rev"=w461:T6)
            n192 = call "Help.About.vi"("SW Version"=w461) -> ()  [unwired: 11 in]
          }
          frame "Simulate OFF", "Simulate ON" {
            n193 = call "Menu.Simulate, Set Menu State.vi"("Menu Tag"=w464, "Menu Ref"=w465) -> ("Sim ON"=w463:bool)  [unwired: 8 in, 1 out]
            n194 = To Variant(anything=w463) -> (Variant=w467:variant)
            n195 = call "Q.Enqueue Task.vi"("Data1"=w467, "Task Name"="Simulate", "Q In"=w468) -> ()  [unwired: 7 in, 2 out]
          }
          frame "Show Block Diagram" {
            n196 = call "Module.Window, Q Task.vi"("Action"=Window.Task,_Action."Open Block Diagram()", "Q In"=w470) -> ()  [unwired: 8 in, 2 out]
          }
          frame "Go to Maint Tab" {
            n197 = call "Module.Window, Q Task.vi"("Action"=Window.Task,_Action."Show Maint Tab(Bool)", "Q In"=w472) -> ()  [unwired: 8 in, 2 out]
          }
        }
      }
      event User Event {
        n198 = event-data() -> ()  [unwired: 1 in, 5 out]
      }
      event "Test Start": Value Change {
        n199 = event-data() -> ()  [unwired: 1 in, 6 out]
        n200 = Send Notification(notification=FALSE, notifier=w474) -> ()  [unwired: 1 in, 2 out]
        n201 = call "Q.Enqueue Seq.vi"("Seq Task Name"="Test Start" ("Task Name"), "Q In"=w476) -> ()  [unwired: 8 in, 2 out]
      }
      event "Test Abort": Value Change {
        n202 = event-data() -> ()  [unwired: 1 in, 6 out]
        n203 = Send Notification(notification=TRUE, notifier=w479) -> ()  [unwired: 1 in, 2 out]
        n204 = call "Q.Enqueue Seq.vi"("Top of Q"=TRUE, "Seq Task Name"="Test Abort" ("Task Name"), "Q In"=w481) -> ()  [unwired: 7 in, 2 out]
      }
      event "Test Reset": Value Change {
        n205 = event-data() -> ()  [unwired: 1 in, 6 out]
        n206 = call "Q.Enqueue Seq.vi"("Seq Task Name"="Test Reset" ("Task Name"), "Q In"=w483) -> ()  [unwired: 8 in, 2 out]
      }
    }
  }
